vi "XYArray from OffsetMultiplier.vi"(2 "Y Scale.Offset and Multiplier":T1, 3 "X Scale.Offset and Multiplier":T1, 4 "Intensity array":dbl[][](array[numeric])) -> (0 "y array":dbl[](array[numeric]), 1 "x array":dbl[](array[numeric]))   [LabVIEW 2016]
uses:
  <vilib>/Utility/miscctls.llb/LVOffsetAndMultiplierTypeDef.ctl
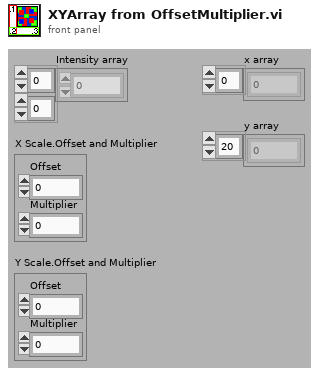
[diagram p1: front panel]
types:
  T1 = typedef "LVOffsetAndMultiplierTypeDef.ctl" = cluster{"Offset":dbl, "Multiplier":dbl}
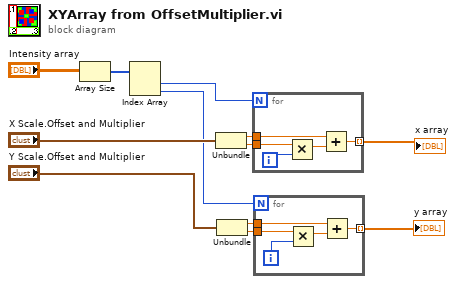
[diagram p0: block diagram]
diagram:
  n1 = Array Size(array="Intensity array") -> (size(s)=w2:i32[])
  n2 = Index Array(array=w2) -> (element #1=w7:i32, element #2=w1:i32)  [unwired: 2 in]
  n3 = Unbundle("X Scale.Offset and Multiplier") -> ("Offset"=w3:dbl, "Multiplier"=w4:dbl)
  n4 = Unbundle("Y Scale.Offset and Multiplier") -> ("Offset"=w6:dbl, "Multiplier"=w5:dbl)
  n5 = for {
    N: w7 -> [_]
    tunnel: w3 -> [w15]
    tunnel: w4 -> [w17]
    tunnel: [w13] -> w11 mode=indexing
    i -> [w16]
    n6 = Multiply(x=w17, y=w16) -> (x*y=w14:dbl)
    n7 = Add(x=w15, y=w14) -> (x+y=w13:dbl)
  }
  "x array" <- w11
  n8 = for {
    N: w1 -> [_]
    tunnel: w6 -> [w20]
    tunnel: w5 -> [w22]
    tunnel: [w18] -> w12 mode=indexing
    i -> [w21]
    n9 = Multiply(x=w22, y=w21) -> (x*y=w19:dbl)
    n10 = Add(x=w20, y=w19) -> (x+y=w18:dbl)
  }
  "y array" <- w12
